vi "Data and Type.vi"(8 "error in (no error)":errorcluster, 11 "Message in":refnum<class "Message.lvclass">) -> (0 "error out":errorcluster, 1 "Format":T1, 2 "Data":string, 3 "Message out":refnum<class "Message.lvclass">)   [LabVIEW 2020, in "Stream-Simple-Msg.lvlib" / "Message.lvclass"]
uses:
  Message.lvclass
  Format.ctl
  Stream-Simple-Msg.lvlib
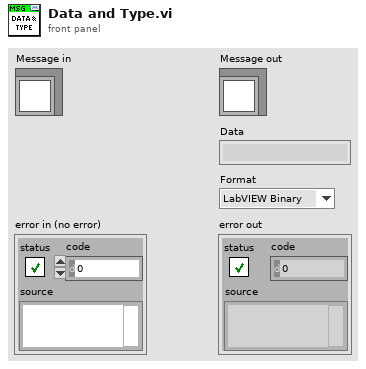
[diagram p1: front panel]
types:
  T1 = typedef "Stream-Simple-Msg.lvlib/Format.ctl" = enum16{"LabVIEW Binary", "JSON"}
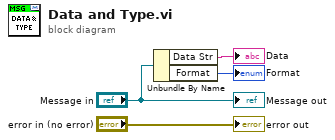
[diagram p0: block diagram]
diagram:
  n1 = Unbundle By Name("Message in") -> ("Data Str"=→"Data":string, "Format"=→"Format":T1)
  "error out" <- "error in (no error)"
  "Message out" <- "Message in"
